vi "Setup.vi"(8 "error in (no error)":errorcluster, 11 "ProjectBase in":refnum<class "Project.lvclass">) -> (0 "error out":errorcluster, 3 "ProjectBase out":refnum<class "Project.lvclass">)   [LabVIEW 2015, in "Project.lvclass"]
uses:
  Project.lvclass
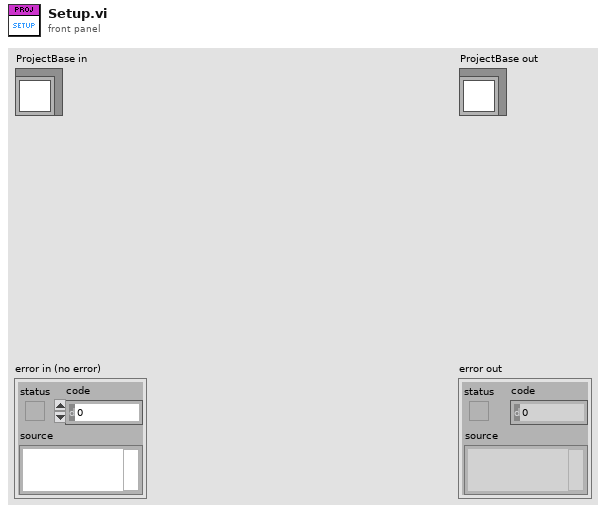
[diagram p1: front panel]
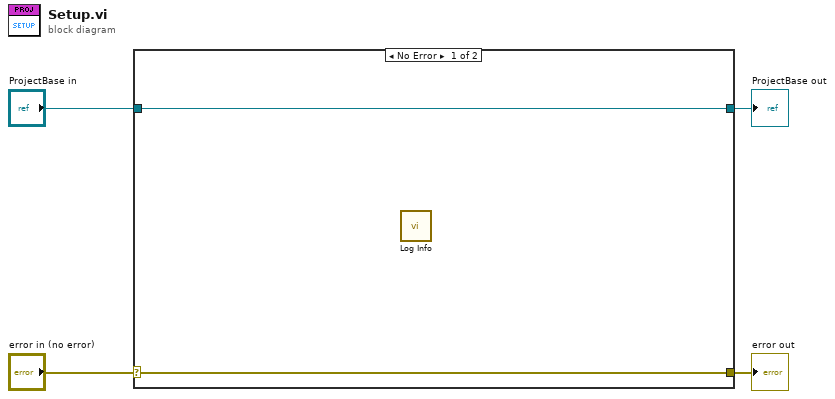
[diagram p0: block diagram]
diagram:
  n1 = case shown="No Error" "error in (no error)" {
    selector: "error in (no error)" -> [w5 w8]
    tunnel: [w5 w8] -> w3
    tunnel: [w6 w7] -> w1
    tunnel: "ProjectBase in" -> [w6 w7]
    frame No Error {
      n2 = call "Log Info.vi"() -> ()  [unwired: 5 in, 1 out]
    }
    frame Error {
    }
  }
  "error out" <- w3
  "ProjectBase out" <- w1
